vi "Report.vi"() -> ()   [LabVIEW 2017]
uses:
  <vilib>/Utility/miscctls.llb/LVRowAndColumnUnsignedTypeDef.ctl
  a160b8e7-0040-4e34-a052-5f80b3aab475.vi
  <vilib>/addons/database/Connection.llb/DB Tools Open Connec (String).vi
  <vilib>/Utility/file.llb/Write Delimited Spreadsheet (string).vi
  Global/Global 1.vi
  <vilib>/regexp/Match Regular Expression.xnode
  <vilib>/addons/database/NI_Database_API.lvlib
  <vilib>/Utility/NIReport.llb/NI_report.lvclass
  <vilib>/Utility/NIReport.llb/Append Text Table to Report (wrap).vi
  <vilib>/Utility/miscctls.llb/LVRowAndColumnTypeDef.ctl
panel:
  out "reposr save header":string[](array[string])
  in  "SELECT REPORT TYPE":string(combo)="WITH TRECIABILITY"
  out "error out":errorcluster
  in  "error in (no error)":errorcluster
  in  "GET REPORT":bool
  in  "EXIT":bool
  in  "EXPORT TO EXCEL":bool
  in  "TO":timestamp format="%<%x>T"
  in  "FROM":timestamp format="%<%x>T"
  in  "BARCODE":string
  in  "TYPE":string(combo)="DATE TIME"
  in  "STATION WISE":string(combo)="0"
  out "Table":string[][](table)
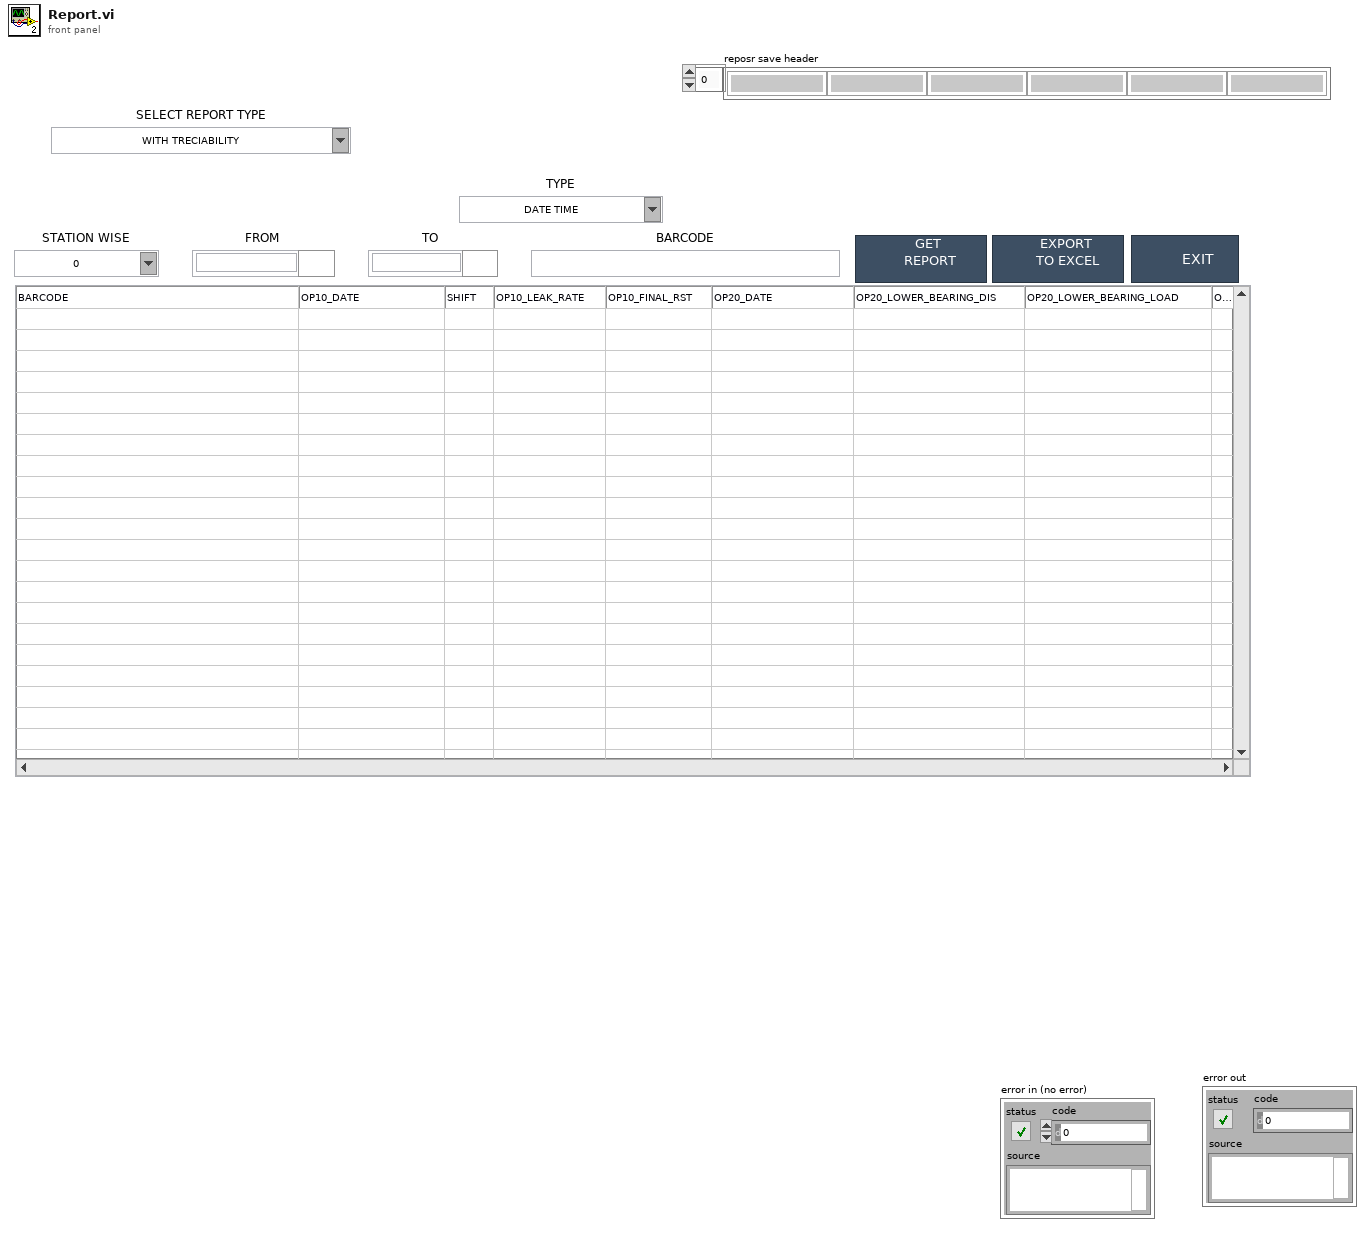
[diagram p1: front panel]
types:
  T1 = typedef "NI_Database_API.lvlib/Conn ObjectReference.ctl" = refnum<k1>
  T2 = typedef "LVRowAndColumnUnsignedTypeDef.ctl" = cluster{"Row":u32, "Column":u32}
  T3 = typedef "LVRowAndColumnTypeDef.ctl" = cluster{"Row":i32, "Column":i32}
  T4 = enum16{"Standard Report", "HTML", "Word", "Excel"}
  T5 = enum16{"maximized", "minimized", "normal", "no change"}
  T6 = enum32{"invalid app kind", "Development System", "Run Time System", "Student Edition", "Embedded LabVIEW", "Evaluation", "Custom"}
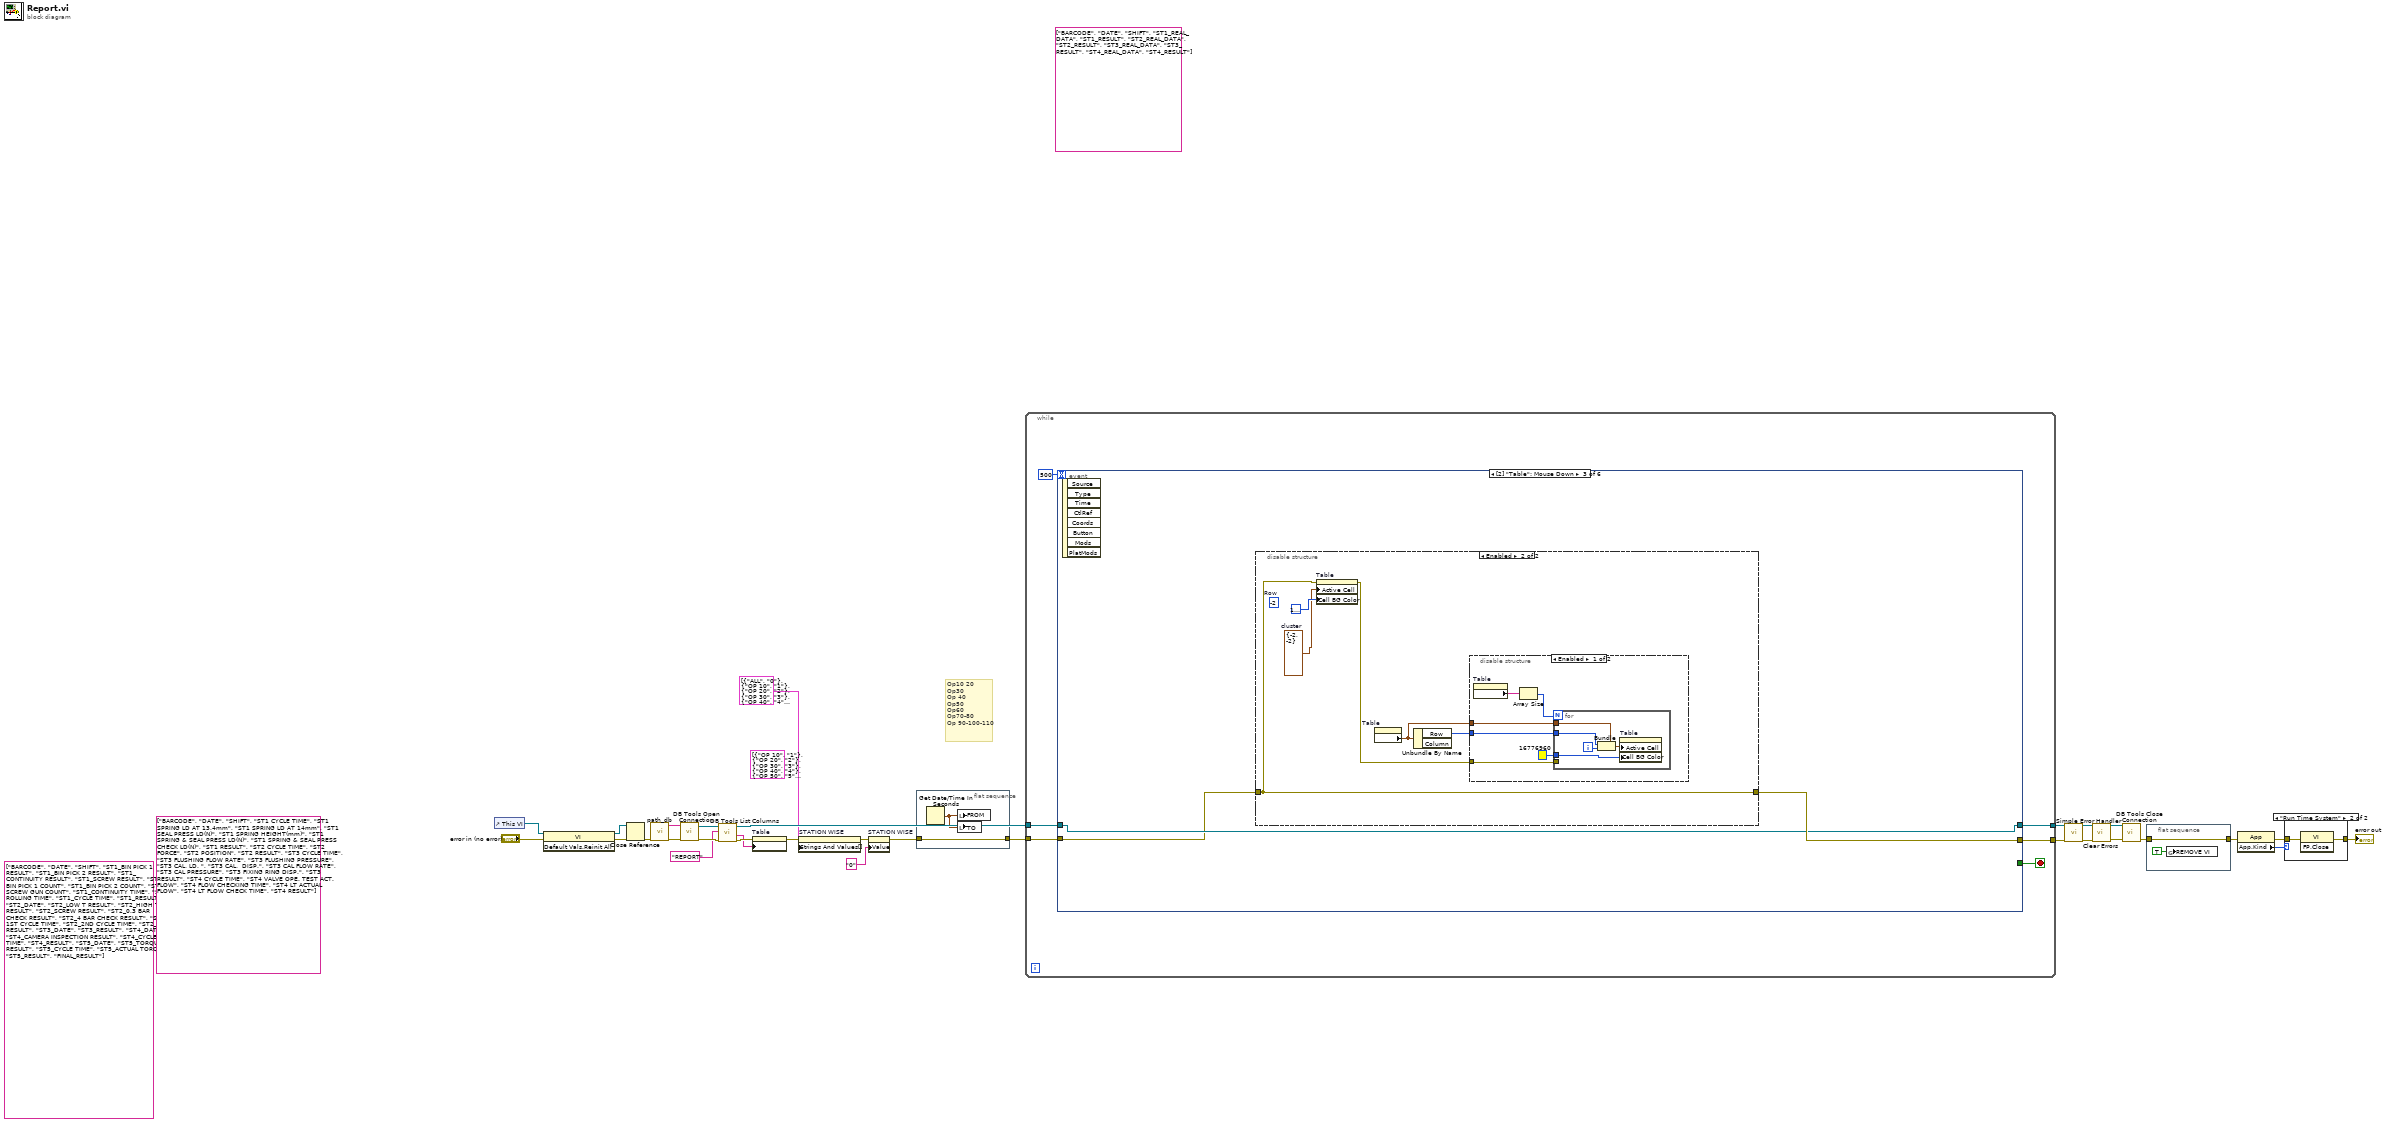
[diagram p0: block diagram]
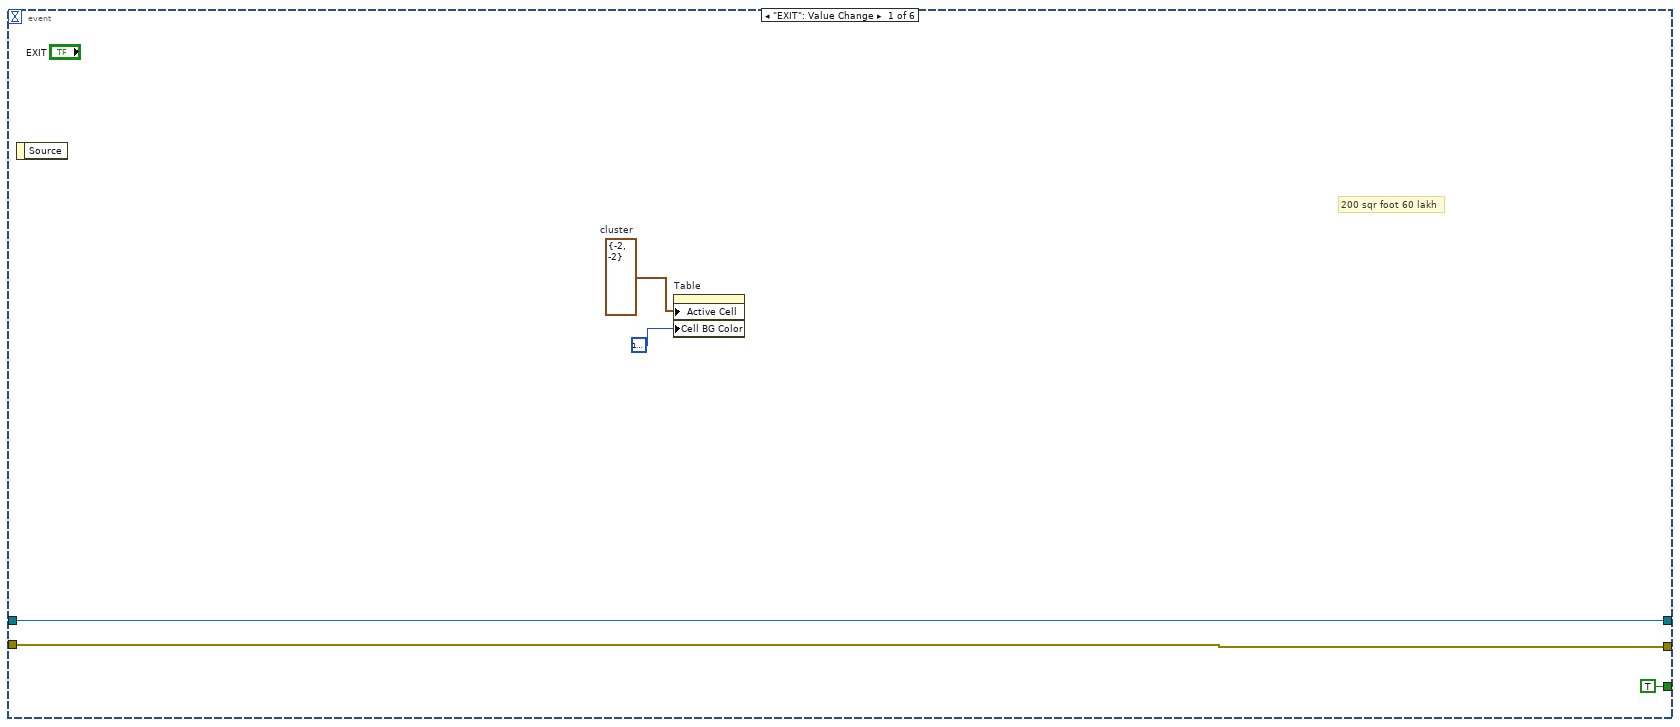
[diagram p2: hidden frame]
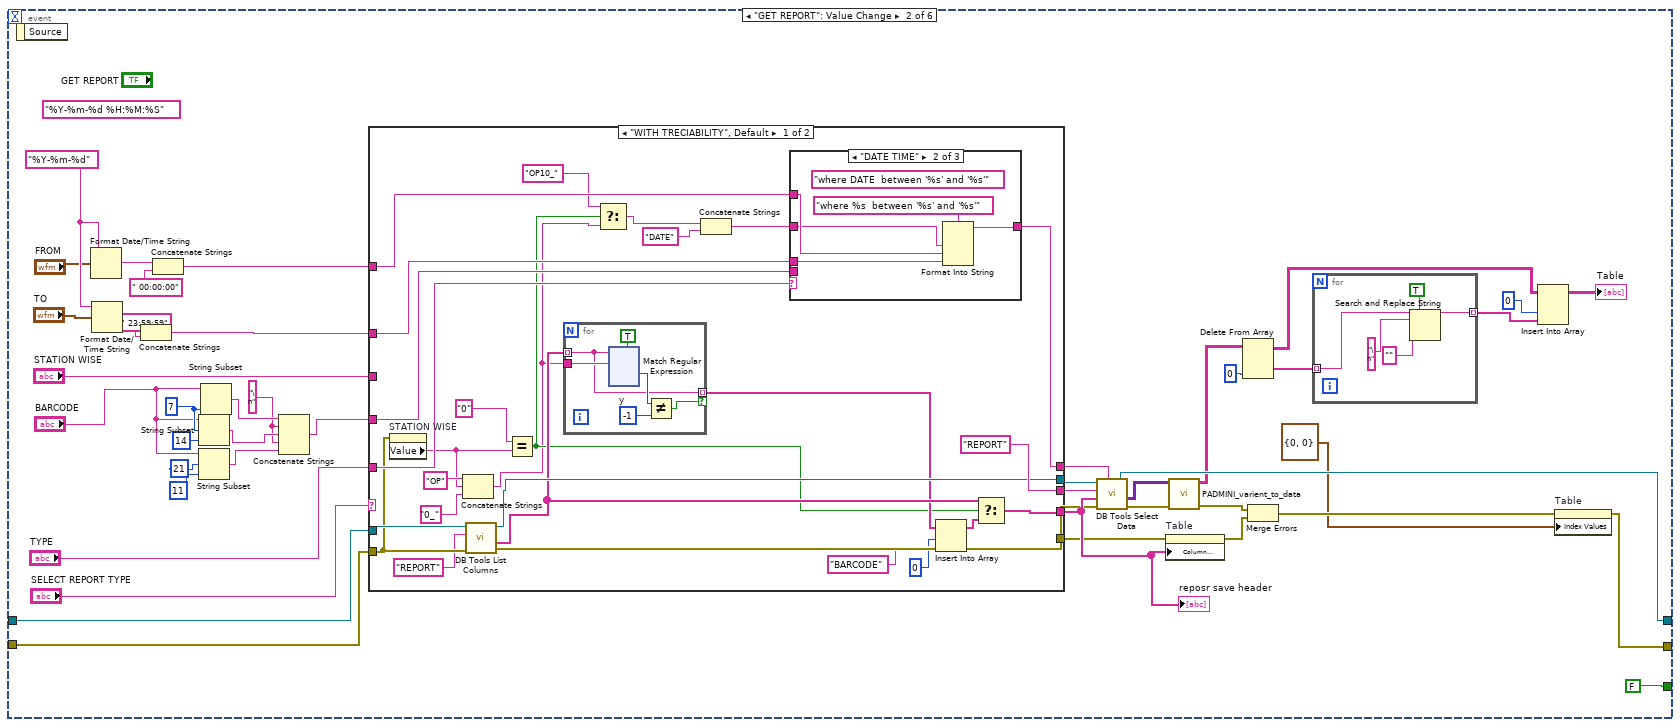
[diagram p3: hidden frame]
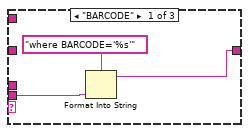
[diagram p4: hidden frame]
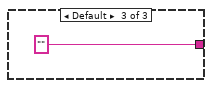
[diagram p5: hidden frame]
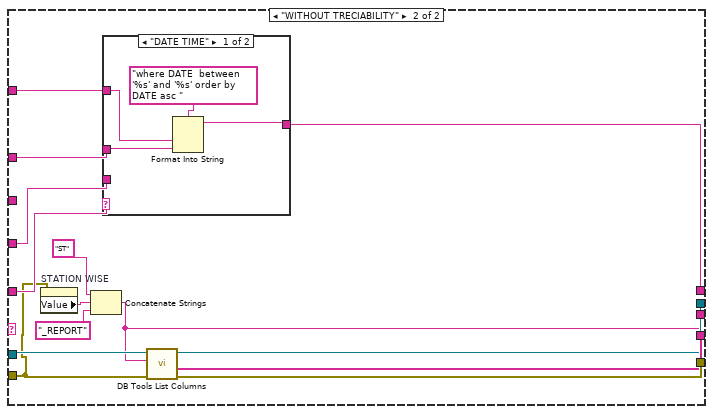
[diagram p6: hidden frame]
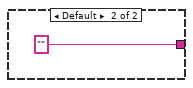
[diagram p7: hidden frame]
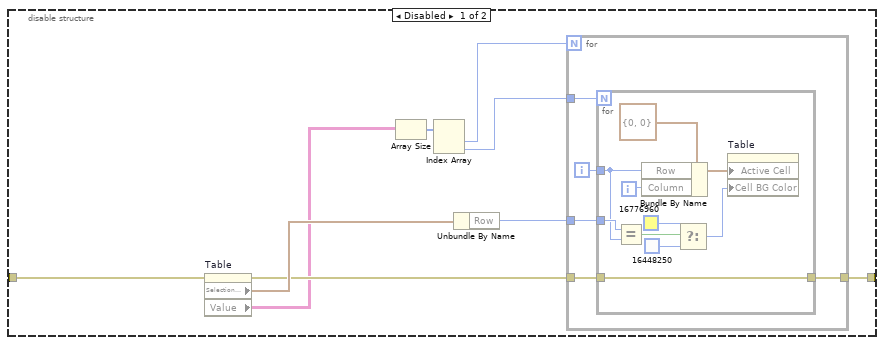
[diagram p8: hidden frame]
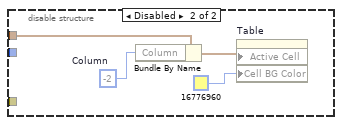
[diagram p9: hidden frame]
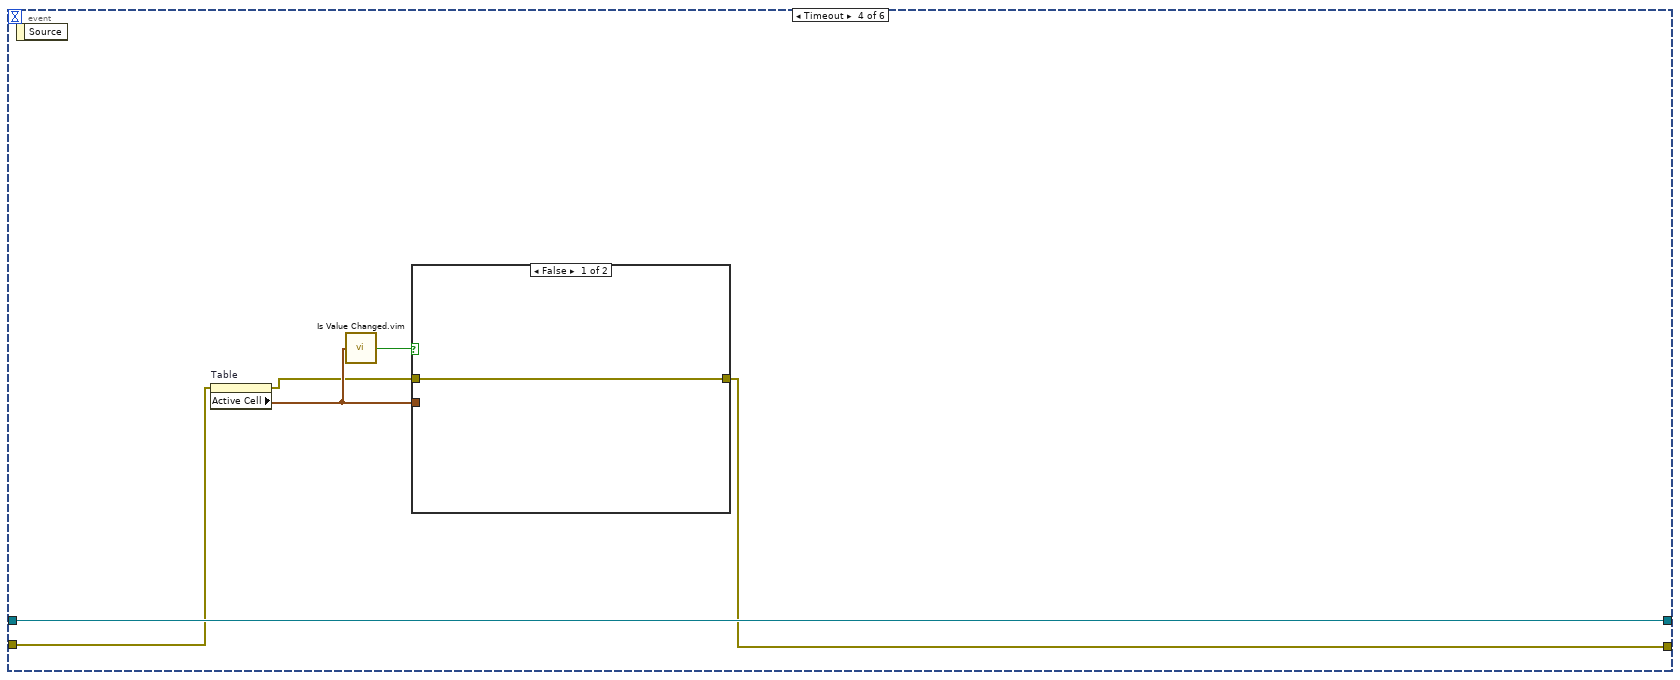
[diagram p10: hidden frame]
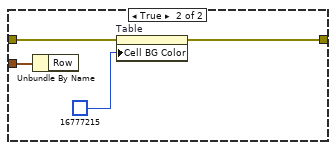
[diagram p11: hidden frame]
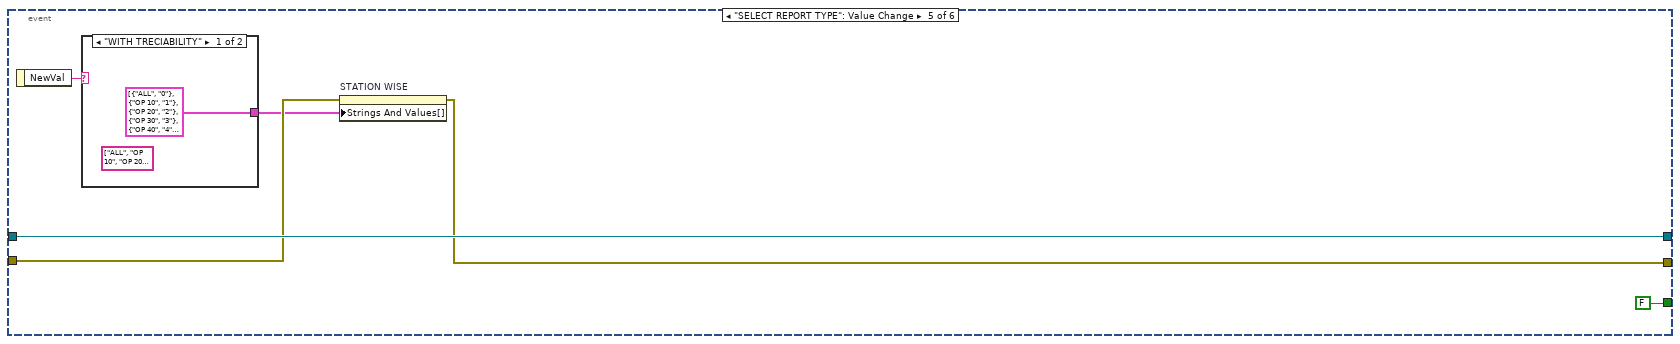
[diagram p12: hidden frame]
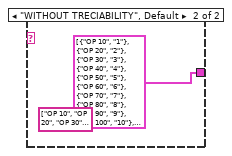
[diagram p13: hidden frame]
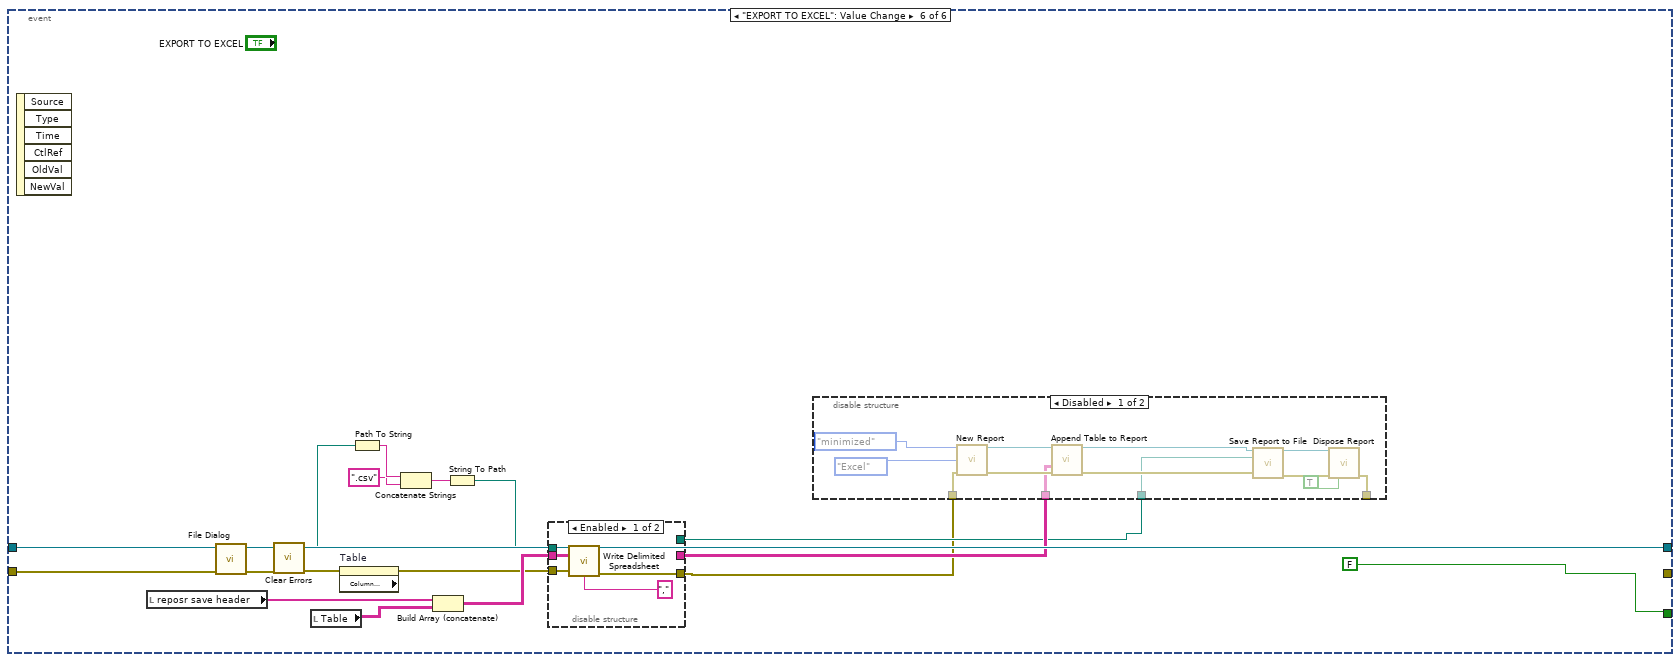
[diagram p14: hidden frame]
diagram:
  (unwired) cluster{"String":string, "Value":string}[] [{"String"="OP 10", "Value"="1"}, {"String"="OP 20", "Value"="2"}, {"String"="OP 30", "Value"="3"}, {"String"="OP 40", "Value"="4"}, {"String"="OP 50", "Value"="5"}, {"String"="OP 60", "Value"="6"}, {"String"="OP 70", "Value"="7"}, {"String"="OP 80", "Value"="8"}, {"String"="OP 90", "Value"="9"}, {"String"="OP 100", "Value"="10"}, {"String"="OP 110", "Value"="11"}] ("Strings And Values [] 2")
  (unwired) string[] ["BARCODE", "DATE", "SHIFT", "ST1_REAL_DATA", "ST1_RESULT", "ST2_REAL_DATA", "ST2_RESULT", "ST3_REAL_DATA", "ST3_RESULT", "ST4_REAL_DATA", "ST4_RESULT"]
  (unwired) string[] ["BARCODE", "DATE", "SHIFT", "ST1_BIN PICK 1 RESULT", "ST1_BIN PICK 2 RESULT", "ST1_CONTINUITY RESULT", "ST1_SCREW RESULT", "ST1_BIN PICK 1 COUNT", "ST1_BIN PICK 2 COUNT", "ST1_SCREW GUN COUNT", "ST1_CONTINUITY TIME", "ST1_ROLLING TIME", "ST1_CYCLE TIME", "ST1_RESULT", "ST2_DATE", "ST2_LOW T RESULT", "ST2_HIGH T RESULT", "ST2_SCREW RESULT", "ST2_0.3 BAR CHECK RESULT", "ST2_4 BAR CHECK RESULT", "ST2_1ST CYCLE TIME", "ST2_2ND CYCLE TIME", "ST2_RESULT", "ST3_DATE", "ST3_RESULT", "ST4_DATE", "ST4_CAMERA INSPECTION RESULT", "ST4_CYCLE TIME", "ST4_RESULT", "ST5_DATE", "ST5_TORQUE RESULT", "ST5_CYCLE TIME", "ST5_ACTUAL TORQUE", "ST5_RESULT", "FINAL_RESULT"]
  (unwired) string[] ["BARCODE", "DATE", "SHIFT", "ST1 CYCLE TIME", "ST1 SPRING LD AT 13.4mm", "ST1 SPRING LD AT 14mm", "ST1 SEAL PRESS LD(N)", "ST1 SPRING HEIGHT(mm)", "ST1 SPRING & SEAL PRESS LD(N)", "ST1 SPRING & SEAL PRESS CHECK LD(N)", "ST1 RESULT", "ST2 CYCLE TIME", "ST2 FORCE", "ST2 POSITION", "ST2 RESULT", "ST3 CYCLE TIME", "ST3 FLUSHING FLOW RATE", "ST3 FLUSHING PRESSURE", "ST3 CAL. LD. ", "ST3 CAL.  DISP.", "ST3 CAL FLOW RATE", "ST3 CAL PRESSURE", "ST3 FIXING RING DISP.", "ST3 RESULT", "ST4 CYCLE TIME", "ST4 VALVE OPE. TEST ACT. FLOW", "ST4 FLOW CHECKING TIME", "ST4 LT ACTUAL FLOW", "ST4 LT FLOW CHECK TIME", "ST4 RESULT"]
  # "Op10 20\nOp30\nOp 40\nOp50\nOp60\nOp70-80\nOp 90-100-110"
  n1 = control-ref of="This VI"() -> (w28:refnum<vi>)
  n2 = invoke class="VI" method="Default Vals.Reinit All"(reference=w28, error in="error in (no error)") -> (reference out=w26:refnum<vi>, error out=w25:errorcluster)  [unwired: 1 in, 1 out]
  n3 = Close Reference(reference=w26, error in (no error)=w25) -> (error out=w16:errorcluster)
  n4 = call "path_db.vi"("error in"=w16) -> ("error out"=w18:errorcluster, "resulting string"=w17:string)  [unwired: 9 in]
  n5 = call-poly <vilib>:"DB Tools Open Connection.vi"("error in (no error)"=w18, "connection information"=w17) -> ("error out"=w11:errorcluster, "connection reference"=w8:T1)  [unwired: 6 in]
  n6 = call <vilib>:"DB Tools List Columns.vi"("error in (no error)"=w11, "table"="REPORT", "connection reference"=w8) -> ("error out"=w10:errorcluster, "columns"=w7:string[], "connection reference out"=w9:T1)  [unwired: 1 in, 1 out]
  n7 = property on="Table" class="Tbl (strict)"(error in=w10, "Column Headers[]"=w7) -> (error out=w13:errorcluster)  [unwired: 1 in, 1 out]
  n8 = property on="STATION WISE" class="CmbBox"(error in=w13, "Strings And Values[]"=cluster{"String":string, "Value":string}[] [{"String"="ALL", "Value"="0"}, {"String"="OP 10", "Value"="1"}, {"String"="OP 20", "Value"="2"}, {"String"="OP 30", "Value"="3"}, {"String"="OP 40", "Value"="4"}, {"String"="OP 50", "Value"="5"}, {"String"="OP 60", "Value"="6"}, {"String"="OP 70", "Value"="7"}, {"String"="OP 80", "Value"="8"}, {"String"="OP 90", "Value"="9"}, {"String"="OP 100", "Value"="10"}, {"String"="OP 110", "Value"="11"}] ("Strings And Values [] 2")) -> (error out=w5:errorcluster)  [unwired: 1 in, 1 out]
  n9 = property on="STATION WISE" class="CmbBox"(error in=w5, "Value"="0") -> (error out=w4:errorcluster)  [unwired: 1 in, 1 out]
  n10 = flat-sequence {
    tunnel: w4 -> [w29]
    tunnel: [w29] -> w12
    frame #0 {
      n11 = Get Date/Time In Seconds() -> (seconds since 1Jan1904=w30:timestamp)
      n12 = local write "FROM"(w30) -> ()
      n13 = local write "TO"(w30) -> ()
    }
  }
  n14 = while {
    tunnel: [w33] -> w1
    tunnel: w12 -> [w35]
    tunnel: w9 -> [w34]
    tunnel: [w32] -> w14
    stop <- w36 stop-if-true
    n15 = event shown="[2] \"Table\": Mouse Down" {
      selector: _ -> [_ _ _ _ _ _]
      dyn-events: _ -> [_ _ _ _ _ _]
      timeout: 500 -> [_ _ _ _ _ _]
      tunnel: [TRUE FALSE _ _ FALSE FALSE] -> w36
      tunnel: w35 -> [w39 w65 w267 w317 w329 w338]
      tunnel: w34 -> [w40 w63 w268 w320 w331 w349]
      tunnel: [w40 w71 w268 w320 w331 w349] -> w32
      tunnel: [w39 w52 w269 w315 w326 _] -> w33
      event "EXIT": Value Change {
        w37 = cluster{"Row":i32, "Row":i32} {"Row"=-2, "Row"=-2}  # cluster
        # "200 sqr foot 60 lakh"
        n16 = event-data() -> ()  [unwired: 1 in, 1 out]
        n17 = property on="Table" class="Tbl (strict)"("Active Cell"=w37, "Cell BG Color"=u32 16777226) -> ()  [unwired: 2 in, 2 out]
      }
      event "GET REPORT": Value Change {
        w44 = "\n"
        w51 = 7 ("line index")
        (unwired) "%Y-%m-%d %H:%M:%S" ("time format string (%c)")
        w84 = "%Y-%m-%d" ("time format string (%c)")
        n18 = event-data() -> ()  [unwired: 1 in, 1 out]
        n19 = Format Date/Time String(time format string (%c)=w84, seconds (now)="FROM") -> (date/time string=w78:string)  [unwired: 1 in]
        n20 = Format Date/Time String(time format string (%c)=w84, seconds (now)="TO") -> (date/time string=w75:string)  [unwired: 1 in]
        n21 = Concatenate Strings(w75, " 23:59:59" ("time format string (%c)")) -> (w74:string)
        n22 = Concatenate Strings(w78, " 00:00:00" ("time format string (%c)")) -> (w77:string)
        n23 = String Subset(string="BARCODE", offset (0)=w51, length (rest)=14 ("line index")) -> (substring=w46:string)
        n24 = String Subset(string="BARCODE", offset (0)=21 ("line index"), length (rest)=11 ("line index")) -> (substring=w45:string)
        n25 = String Subset(string="BARCODE", length (rest)=w51) -> (substring=w47:string)  [unwired: 1 in]
        n26 = Concatenate Strings(w47, w44, w46, w44, w45) -> (w43:string)
        n27 = case shown="\"WITH TRECIABILITY\", Default" "SELECT REPORT TYPE" {
          tunnel: "TYPE" -> [w118 w261]
          tunnel: [w117 w260] -> w85
          tunnel: w43 -> [w116 w259]
          tunnel: w77 -> [w115 w258]
          tunnel: w74 -> [w100 w254]
          tunnel: "STATION WISE" -> [_ _]
          tunnel: ["REPORT" w249] -> w66
          tunnel: w65 -> [w106 w248]
          tunnel: [w111 w253] -> w60
          tunnel: [w98 w252] -> w64
          tunnel: w63 -> [w113 w251]
          tunnel: [w112 w250] -> w62
          frame "WITH TRECIABILITY", Default {
            n28 = property on="STATION WISE" class="CmbBox"(error in=w106) -> ("Value"=w101:string)  [unwired: 1 in, 2 out]
            n29 = Concatenate Strings("OP" ("element"), w101, "0_" ("element")) -> (w93:string)
            n30 = call <vilib>:"DB Tools List Columns.vi"("error in (no error)"=w106, "table"="REPORT", "connection reference"=w113) -> ("error out"=w111:errorcluster, "columns"=w105:string[], "connection reference out"=w112:T1)  [unwired: 1 in, 1 out]
            n31 = Equal?(x="0", y=w101) -> (x = y?=w95:bool)
            n32 = for {
              tunnel: w105 -> [w120] mode=indexing
              tunnel: w93 -> [w124]
              tunnel: [w120] -> w99 mode=indexing if=w119
              w121 = -1  # y
              n33 = xnode "Match Regular Expression"("input string"=w120, "regular expression"=w124, "multiline? (F)"=TRUE) -> ("offset past match"=w122:i32)  [unwired: 3 in, 4 out]
              n34 = Not Equal?(x=w122, y=w121) -> (x != y?=w119:bool)
            }
            n35 = Select(t="OP10_", s=w95, f=w93) -> (s? t:f=w92:string)
            n36 = Concatenate Strings(w92, "DATE") -> (w96:string)
            n37 = case shown="\"DATE TIME\"" w118 {
              tunnel: [w240 w245 ""] -> w117
              tunnel: w116 -> [w239 _ _]
              tunnel: w115 -> [_ w244 _]
              tunnel: w100 -> [_ w243 _]
              tunnel: w96 -> [_ w242 _]
              frame "BARCODE" {
                n38 = Format Into String(format string="where BARCODE='%s'", w239) -> (resulting string=w240:string)  [unwired: 2 in, 1 out]
              }
              frame "DATE TIME" {
                (unwired) "where DATE  between '%s' and '%s'"
                n39 = Format Into String(format string="where %s  between '%s' and '%s'", w242, w244, w243) -> (resulting string=w245:string)  [unwired: 2 in, 1 out]
              }
              frame Default {
              }
            }
            n40 = Insert Into Array(array=w99, index=0, new element="BARCODE" ("String")) -> (w109:string[])
            n41 = Select(t=w105, s=w95, f=w109) -> (s? t:f=w98:string[])
          }
          frame "WITHOUT TRECIABILITY" {
            n42 = property on="STATION WISE" class="CmbBox"(error in=w248) -> ("Value"=w257:string)  [unwired: 1 in, 2 out]
            n43 = Concatenate Strings("ST", w257, "_REPORT") -> (w249:string)
            n44 = case shown="\"DATE TIME\"" w261 {
              tunnel: [w265 ""] -> w260
              tunnel: w259 -> [_ _]
              tunnel: w258 -> [w264 _]
              tunnel: w254 -> [w263 _]
              frame "DATE TIME" {
                n45 = Format Into String(format string="where DATE  between '%s' and '%s' order by DATE asc ", w264, w263) -> (resulting string=w265:string)  [unwired: 2 in, 1 out]
              }
              frame Default {
              }
            }
            n46 = call <vilib>:"DB Tools List Columns.vi"("error in (no error)"=w248, "table"=w249, "connection reference"=w251) -> ("error out"=w253:errorcluster, "columns"=w252:string[], "connection reference out"=w250:T1)  [unwired: 1 in, 1 out]
          }
        }
        "reposr save header" <- w64
        n47 = call <vilib>:"DB Tools Select Data.vi"("condition"=w85, "error in (no error)"=w60, "columns"=w64, "table"=w66, "connection reference"=w62) -> ("error out"=w69:errorcluster, "data"=w73:variant[][], "connection reference out"=w71:T1)  [unwired: 1 in]
        n48 = property on="Table" class="Tbl (strict)"(error in=w60, "Column Headers[]"=w64) -> (error out=w68:errorcluster)  [unwired: 1 in, 1 out]
        n49 = call "PADMINI_varient_to_data.vi"("error in (no error)"=w69, "data"=w73) -> ("error out"=w67:errorcluster, "Array"=w55:string[][])  [unwired: 8 in]
        n50 = Delete From Array(array=w55, index (col)=0 ("disabled index (col)")) -> (deleted portion=w58:string[], array with subset deleted=w56:string[][])  [unwired: 2 in]
        n51 = Merge Errors(w67, w68) -> (w72:errorcluster)
        n52 = for {
          tunnel: w58 -> [w88] mode=indexing
          tunnel: [w87] -> w57 mode=indexing
          n53 = Search and Replace String(replace all?=TRUE ("replace all? (F)"), input string=w88, search string="\n", replace string="" ("replace string (\"\")")) -> (result string=w87:string)  [unwired: 4 in, 3 out]
        }
        n54 = Insert Into Array(array=w56, index (col)=0 ("disabled index (col)"), new element=w57) -> (→"Table":string[][])  [unwired: 1 in]
        n55 = property on="Table" class="Tbl (strict)"(error in=w72, "Index Values"=T2 {"Row"=0, "Column"=0}) -> (error out=w52:errorcluster)  [unwired: 1 in, 1 out]
      }
      event "Table": Mouse Down {
        n56 = event-data() -> ()  [unwired: 1 in, 8 out]
        n57 = disable-structure shown="Enabled" {
          disable-tunnel: [w278 w295] -> w269
          disable-tunnel: w267 -> [w275 w295]
          frame Disabled {
            n58 = property on="Table" class="Tbl (strict)"(error in=w275) -> (error out=w274:errorcluster, "Selection Start"=w276:T3, "Value"=w272:string[][])  [unwired: 1 in, 1 out]
            n59 = Array Size(array=w272) -> (size(s)=w273:i32[])
            n60 = Index Array(array=w273) -> (element #1=w270:i32, element #2=w271:i32)  [unwired: 2 in]
            n61 = Unbundle By Name(w276) -> ("Row"=w277:i32)
            n62 = for {
              N: w270 -> [_]
              tunnel: w277 -> [w281]
              tunnel: w271 -> [w283]
              tunnel: [w279] -> w278
              tunnel: w274 -> [w280]
              i -> [w282]
              n63 = for {
                N: w283 -> [_]
                tunnel: w282 -> [w289]
                tunnel: w281 -> [w290]
                tunnel: w280 -> [w284]
                tunnel: [w284] -> w279
                i -> [w291]
                n64 = Equal?(x=w290, y=w289) -> (x = y?=w288:bool)
                n65 = Bundle By Name(cluster=T3 {"Row"=0, "Column"=0} ("Selection Start 2"), "Row"=w289, "Column"=w291) -> (w292:T3)
                n66 = Select(t=u32 16776960, s=w288, f=u32 16448250) -> (s? t:f=w285:u32)
                n67 = property on="Table" class="Tbl (strict)"("Active Cell"=w292, "Cell BG Color"=w285) -> ()  [unwired: 2 in, 2 out]
              }
            }
          }
          frame Enabled {
            w294 = cluster{"Row":i32, "Row":i32} {"Row"=-2, "Row"=-2}  # cluster
            (unwired) -2  # Row
            n68 = property on="Table" class="Tbl (strict)"(error in=w295, "Active Cell"=w294, "Cell BG Color"=u32 16777226) -> (error out=w296:errorcluster)  [unwired: 1 in, 1 out]
            n69 = property on="Table" class="Tbl (strict)"() -> ("Selection Start"=w297:T3)  [unwired: 2 in, 2 out]
            n70 = Unbundle By Name(w297) -> ("Row"=w299:i32)  [unwired: 1 out]
            n71 = disable-structure shown="Enabled" {
              disable-tunnel: w299 -> [w304 _]
              disable-tunnel: w297 -> [w303 w312]
              disable-tunnel: w296 -> [w300 _]
              frame Enabled {
                n72 = property on="Table" class="Tbl (strict)"() -> ("Column Headers[]"=w302:string[])  [unwired: 2 in, 2 out]
                n73 = Array Size(array=w302) -> (size(s)=w301:i32)
                n74 = for {
                  N: w301 -> [_]
                  tunnel: u32 16776960 -> [w310]
                  tunnel: w303 -> [w309]
                  tunnel: w304 -> [w308]
                  tunnel: w300 -> [_]
                  i -> [w307]
                  n75 = Bundle(cluster=w309, "Row"=w308, "Column"=w307) -> (w306:T3)
                  n76 = property on="Table" class="Tbl (strict)"("Active Cell"=w306, "Cell BG Color"=w310) -> ()  [unwired: 2 in, 2 out]
                }
              }
              frame Disabled {
                w311 = -2  # Column
                n77 = Bundle By Name(cluster=w312, "Column"=w311) -> (w313:T3)
                n78 = property on="Table" class="Tbl (strict)"("Active Cell"=w313, "Cell BG Color"=u32 16776960) -> ()  [unwired: 2 in, 2 out]
              }
            }
          }
        }
      }
      event Timeout {
        n79 = event-data() -> ()  [unwired: 1 in, 1 out]
        n80 = property on="Table" class="Tbl (strict)"(error in=w317) -> (error out=w316:errorcluster, "Active Cell"=w319:T3)  [unwired: 1 in, 1 out]
        n81 = call "Is Value Changed.vim"("value"=w319) -> ("changed or first call?"=w318:bool)
        n82 = case shown="False" w318 {
          tunnel: w319 -> [_ w325]
          tunnel: w316 -> [w321 w323]
          tunnel: [w321 w322] -> w315
          frame False {
          }
          frame True {
            n83 = Unbundle By Name(w325) -> ()  [unwired: 1 out]
            n84 = property on="Table" class="Tbl (strict)"(error in=w323, "Cell BG Color"=u32 16777215) -> (error out=w322:errorcluster)  [unwired: 1 in, 1 out]
          }
        }
      }
      event "SELECT REPORT TYPE": Value Change {
        n85 = event-data() -> ("NewVal"=w330:string)  [unwired: 1 in]
        n86 = case shown="\"WITH TRECIABILITY\"" w330 {
          tunnel: [cluster{"String":string, "Value":string}[] [{"String"="ALL", "Value"="0"}, {"String"="OP 10", "Value"="1"}, {"String"="OP 20", "Value"="2"}, {"String"="OP 30", "Value"="3"}, {"String"="OP 40", "Value"="4"}, {"String"="OP 50", "Value"="5"}, {"String"="OP 60", "Value"="6"}, {"String"="OP 70", "Value"="7"}, {"String"="OP 80", "Value"="8"}, {"String"="OP 90", "Value"="9"}, {"String"="OP 100", "Value"="10"}, {"String"="OP 110", "Value"="11"}] ("Strings And Values [] 2") cluster{"String":string, "Value":string}[] [{"String"="OP 10", "Value"="1"}, {"String"="OP 20", "Value"="2"}, {"String"="OP 30", "Value"="3"}, {"String"="OP 40", "Value"="4"}, {"String"="OP 50", "Value"="5"}, {"String"="OP 60", "Value"="6"}, {"String"="OP 70", "Value"="7"}, {"String"="OP 80", "Value"="8"}, {"String"="OP 90", "Value"="9"}, {"String"="OP 100", "Value"="10"}, {"String"="OP 110", "Value"="11"}] ("Strings And Values [] 2")] -> w327
          frame "WITH TRECIABILITY" {
            (unwired) string[] ["ALL", "OP 10", "OP 20", "OP 30", "OP 40", "OP 50", "OP 60", "OP 70", "OP 80", "OP 90", "OP 100", "OP 110"] ("Strings []")
          }
          frame "WITHOUT TRECIABILITY", Default {
            (unwired) string[] ["OP 10", "OP 20", "OP 30", "OP 40", "OP 50", "OP 60", "OP 70", "OP 80", "OP 90", "OP 100", "OP 110"] ("Strings []")
          }
        }
        n87 = property on="STATION WISE" class="CmbBox"(error in=w329, "Strings And Values[]"=w327) -> (error out=w326:errorcluster)  [unwired: 1 in, 1 out]
      }
      event "EXPORT TO EXCEL": Value Change {
        n88 = event-data() -> ()  [unwired: 1 in, 6 out]
        n89 = local read "reposr save header"() -> (w334:string[])
        n90 = call "File Dialog"("error in"=w338) -> ("selected path"=w347:path, "error out"=w348:errorcluster)  [unwired: 11 in, 2 out]
        n91 = call <vilib>:"Clear Errors.vi"("error in (no error)"=w348) -> ("error out"=w341:errorcluster)  [unwired: 5 in, 1 out]
        n92 = local read "Table"() -> (w350:string[][])
        n93 = property on="Table" class="Tbl (strict)" props=["Column Headers[]"](error in=w341) -> (error out=w340:errorcluster)  [unwired: 1 in, 2 out]
        n94 = Path To String(path=w347) -> (string=w346:string)
        n95 = Concatenate Strings(w346, ".csv" ("string")) -> (w344:string)
        n96 = Build Array (concatenate)(w334, w350) -> (w342:string[][])
        n97 = String To Path(string=w344) -> (path=w343:path)
        n98 = disable-structure shown="Enabled" {
          disable-tunnel: w343 -> [w369 w370]
          disable-tunnel: [w368 w372] -> w335
          disable-tunnel: w342 -> [w367 w371]
          disable-tunnel: w340 -> [w365 w372]
          disable-tunnel: [_ w371] -> w337
          disable-tunnel: [_ w370] -> w336
          frame Enabled {
            n99 = call-poly <vilib>:"Write Delimited Spreadsheet.vi"("file path (dialog if empty)"=w369, "2D data"=w367, "error in (no error)"=w365, "delimiter (\\t)"="," ("delimiter (\\t)")) -> ("error out"=w368:errorcluster)  [unwired: 10 in, 1 out]
          }
          frame Disabled {
          }
        }
        n100 = disable-structure shown="Disabled" {
          disable-tunnel: w337 -> [w354 _]
          disable-tunnel: w336 -> [w353 _]
          disable-tunnel: [w352 w364] -> _
          disable-tunnel: w335 -> [w351 w364]
          frame Disabled {
            n101 = call <vilib>:"New Report.vi"("window state (normal)"=T5."minimized", "report type"=T4."Excel", "error in (no error)"=w351) -> ("report out"=w361:refnum<class "NI_report.lvclass">, "error out"=w360:errorcluster)  [unwired: 11 in]
            n102 = call-poly <vilib>:"Append Table to Report.vi"("report in"=w361, "text data"=w354, "error in (no error)"=w360) -> ("report out"=w357:refnum<class "NI_report.lvclass">, "error out"=w359:errorcluster)  [unwired: 9 in, 2 out]
            n103 = call-dynamic "Save Report to File.vi"("report in"=w357, "report file path"=w353, "error in (no error)"=w359) -> ("report out"=w356:refnum<class "NI_report.lvclass">, "error out"=w358:errorcluster)  [unwired: 11 in]
            n104 = call-dynamic "Dispose Report.vi"("report in"=w356, "error in (no error)"=w358, "close report? (T)"=TRUE) -> ("error out"=w352:errorcluster)  [unwired: 12 in]
          }
          frame Enabled {
          }
        }
      }
    }
  }
  n105 = call <vilib>:"Simple Error Handler.vi"("error in (no error)"=w1) -> ("error out"=w24:errorcluster)  [unwired: 4 in, 4 out]
  n106 = call <vilib>:"Clear Errors.vi"("error in (no error)"=w24) -> ("error out"=w23:errorcluster)  [unwired: 5 in, 1 out]
  n107 = call <vilib>:"DB Tools Close Connection.vi"("error in (no error)"=w23, "connection reference"=w14) -> ("error out"=w15:errorcluster)  [unwired: 5 in]
  n108 = flat-sequence {
    tunnel: [w374] -> w22
    tunnel: w15 -> [w374]
    frame #0 {
      n109 = global write "Global 1.vi" "REMOVE VI"(TRUE ("REMOVE VI")) -> ()
    }
  }
  n110 = property class="App"(error in=w22) -> (error out=w21:errorcluster, "App.Kind"=w20:T6)  [unwired: 1 in, 1 out]
  n111 = case shown="\"Run Time System\"" w20 {
    tunnel: w21 -> [w375 w377]
    tunnel: [w375 w376] -> w19
    frame "Development System", Default {
    }
    frame "Run Time System" {
      n112 = invoke class="VI" method="FP.Close"(error in=w377) -> (error out=w376:errorcluster)  [unwired: 2 in, 2 out]
    }
  }
  "error out" <- w19
